vi "receiveData.vi"(8 "error in (no error)":errorcluster, 11 "ILC in":refnum<class "ILC.lvclass">) -> (0 "error out":errorcluster, 3 "ILC out":refnum<class "ILC.lvclass">)   [LabVIEW 2013, in "ILCCommon.lvlib" / "ILC.lvclass"]
uses:
  <userlib>/Common/ILC/ILC/ILC.lvclass
  <userlib>/Common/ILC/ILC/ILC.lvclass/ILC.ctl
  <userlib>/Common/SerialProtocols/SerialCommunicator/SerialCommunicator.lvclass
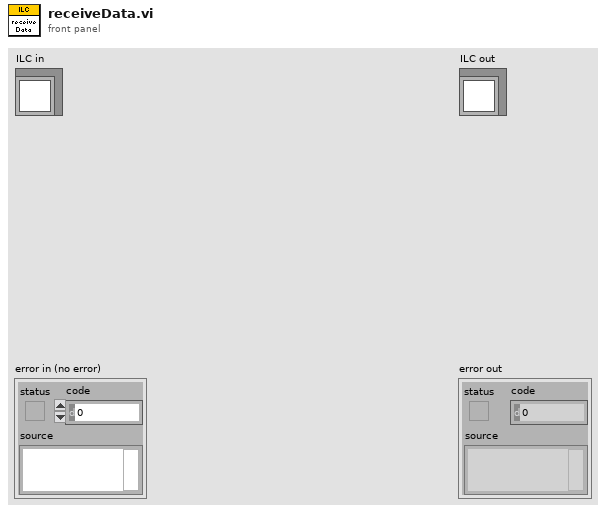
[diagram p1: front panel]
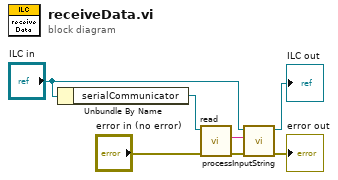
[diagram p0: block diagram]
diagram:
  n1 = Unbundle By Name("ILC in") -> ("serialCommunicator"=w5:refnum<class "SerialCommunicator.lvclass">)
  n2 = call-dynamic "read.vi"("error in (no error)"="error in (no error)", "SerialCommunicator in"=w5) -> ("error out"=w6:errorcluster, "stringRead"=w7:string)  [unwired: 7 in, 1 out]
  n3 = call <userlib>:"processInputString.vi"("error in (no error)"=w6, "stringRead"=w7, "ILC in"="ILC in") -> ("error out"=→"error out":errorcluster, "ILC out"=→"ILC out":refnum<class "ILC.lvclass">)  [unwired: 7 in]
